vi "Events.vi"(8 "counter":i32, 11 "responsein":string) -> (3 "responseout":string)   [LabVIEW 2014]
doc: "Parse a JSONRPC 2.0 string and invokes the corresponding method."
panel:
  # "Events"
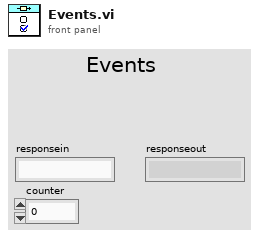
[diagram p1: front panel]
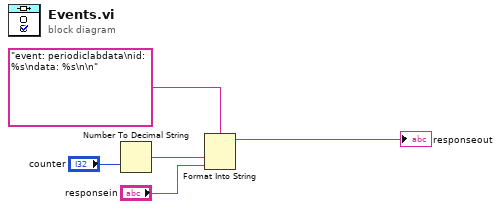
[diagram p0: block diagram]
diagram:
  n1 = Number To Decimal String(number="counter") -> (decimal integer string=w5:string)  [unwired: 1 in]
  n2 = Format Into String(format string="event: periodiclabdata\nid: %s\ndata: %s\n\n", w5, "responsein") -> (resulting string=→"responseout":string)  [unwired: 2 in, 1 out]
